vi "attoDllErrorHandler.vi"(6 "response":string, 9 "error in":errorcluster, 11 "rc":i32) -> (1 "error out":errorcluster)   [LabVIEW 2016]
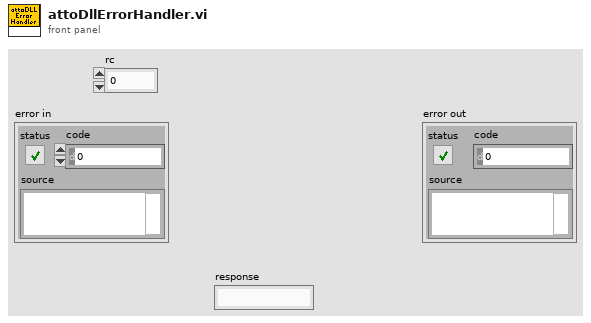
[diagram p1: front panel]
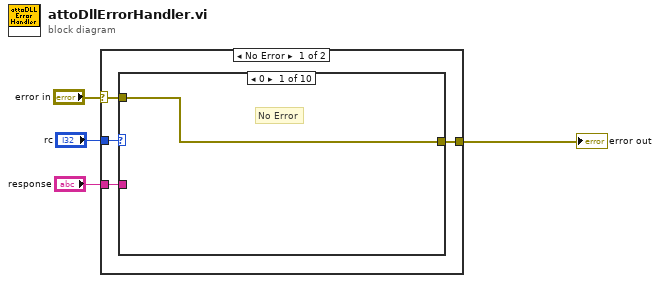
[diagram p0: block diagram]
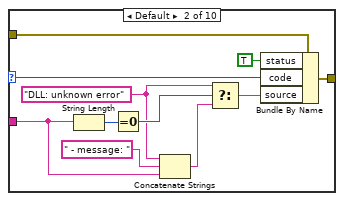
[diagram p2: hidden frame]
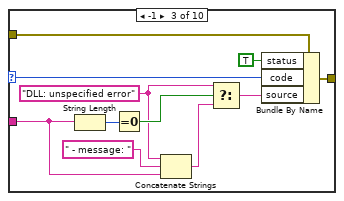
[diagram p3: hidden frame]
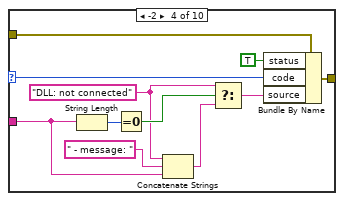
[diagram p4: hidden frame]
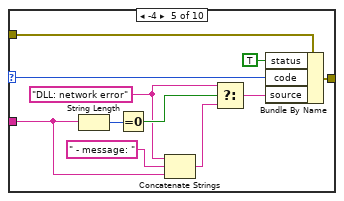
[diagram p5: hidden frame]
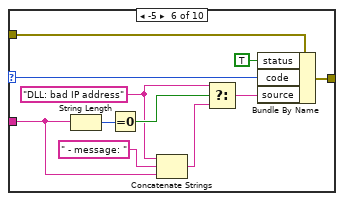
[diagram p6: hidden frame]
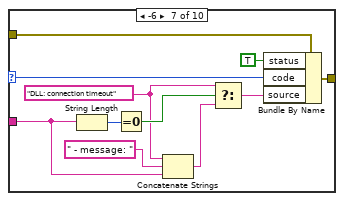
[diagram p7: hidden frame]
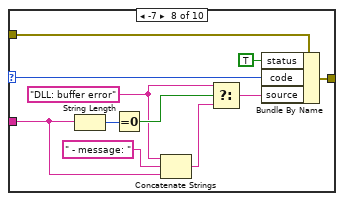
[diagram p8: hidden frame]
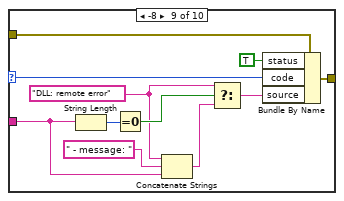
[diagram p9: hidden frame]
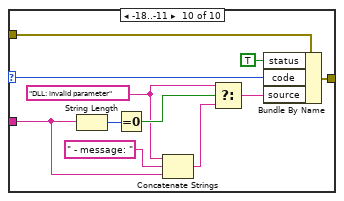
[diagram p10: hidden frame]
diagram:
  n1 = case shown="No Error" "error in" {
    selector: "error in" -> [w6 w109]
    tunnel: "rc" -> [w8 _]
    tunnel: [w7 w109] -> w2
    tunnel: "response" -> [w5 _]
    frame No Error {
      n2 = case shown="0" w8 {
        selector: w8 -> [_ w13 w24 w35 w46 w62 w65 w79 w90 w101]
        tunnel: [w9 w11 w22 w33 w44 w61 w69 w76 w88 w98] -> w7
        tunnel: w6 -> [w9 w14 w25 w36 w47 w63 w68 w80 w91 w102]
        tunnel: w5 -> [_ w12 w23 w34 w45 w56 w66 w78 w89 w100]
        frame 0 {
          # "No Error"
        }
        frame Default {
          w10 = "DLL: unknown error"
          n3 = String Length(string=w12) -> (length=w19:i32)
          n4 = Equal To 0?(x=w19) -> (x = 0?=w17:bool)
          n5 = Concatenate Strings(w10, " - message: " ("string"), w12) -> (w15:string)
          n6 = Select(t=w10, s=w17, f=w15) -> (s? t:f=w16:string)
          n7 = Bundle By Name(cluster=w14, "status"=TRUE, "code"=w13, "source"=w16) -> (w11:errorcluster)
        }
        frame -1 {
          w21 = "DLL: unspecified error"
          n8 = String Length(string=w23) -> (length=w30:i32)
          n9 = Equal To 0?(x=w30) -> (x = 0?=w28:bool)
          n10 = Concatenate Strings(w21, " - message: " ("string"), w23) -> (w26:string)
          n11 = Select(t=w21, s=w28, f=w26) -> (s? t:f=w27:string)
          n12 = Bundle By Name(cluster=w25, "status"=TRUE, "code"=w24, "source"=w27) -> (w22:errorcluster)
        }
        frame -2 {
          w32 = "DLL: not connected"
          n13 = String Length(string=w34) -> (length=w41:i32)
          n14 = Equal To 0?(x=w41) -> (x = 0?=w39:bool)
          n15 = Concatenate Strings(w32, " - message: " ("string"), w34) -> (w37:string)
          n16 = Select(t=w32, s=w39, f=w37) -> (s? t:f=w38:string)
          n17 = Bundle By Name(cluster=w36, "status"=TRUE, "code"=w35, "source"=w38) -> (w33:errorcluster)
        }
        frame -4 {
          w43 = "DLL: network error"
          n18 = String Length(string=w45) -> (length=w52:i32)
          n19 = Equal To 0?(x=w52) -> (x = 0?=w50:bool)
          n20 = Concatenate Strings(w43, " - message: " ("string"), w45) -> (w48:string)
          n21 = Select(t=w43, s=w50, f=w48) -> (s? t:f=w49:string)
          n22 = Bundle By Name(cluster=w47, "status"=TRUE, "code"=w46, "source"=w49) -> (w44:errorcluster)
        }
        frame -5 {
          w57 = "DLL: bad IP address"
          n23 = String Length(string=w56) -> (length=w60:i32)
          n24 = Equal To 0?(x=w60) -> (x = 0?=w58:bool)
          n25 = Concatenate Strings(w57, " - message: " ("string"), w56) -> (w54:string)
          n26 = Select(t=w57, s=w58, f=w54) -> (s? t:f=w55:string)
          n27 = Bundle By Name(cluster=w63, "status"=TRUE, "code"=w62, "source"=w55) -> (w61:errorcluster)
        }
        frame -6 {
          w67 = "DLL: connection timeout"
          n28 = String Length(string=w66) -> (length=w74:i32)
          n29 = Equal To 0?(x=w74) -> (x = 0?=w72:bool)
          n30 = Concatenate Strings(w67, " - message: " ("string"), w66) -> (w70:string)
          n31 = Select(t=w67, s=w72, f=w70) -> (s? t:f=w71:string)
          n32 = Bundle By Name(cluster=w68, "status"=TRUE, "code"=w65, "source"=w71) -> (w69:errorcluster)
        }
        frame -7 {
          w77 = "DLL: buffer error"
          n33 = String Length(string=w78) -> (length=w85:i32)
          n34 = Equal To 0?(x=w85) -> (x = 0?=w83:bool)
          n35 = Concatenate Strings(w77, " - message: " ("string"), w78) -> (w81:string)
          n36 = Select(t=w77, s=w83, f=w81) -> (s? t:f=w82:string)
          n37 = Bundle By Name(cluster=w80, "status"=TRUE, "code"=w79, "source"=w82) -> (w76:errorcluster)
        }
        frame -8 {
          w87 = "DLL: remote error"
          n38 = String Length(string=w89) -> (length=w96:i32)
          n39 = Equal To 0?(x=w96) -> (x = 0?=w94:bool)
          n40 = Concatenate Strings(w87, " - message: " ("string"), w89) -> (w92:string)
          n41 = Select(t=w87, s=w94, f=w92) -> (s? t:f=w93:string)
          n42 = Bundle By Name(cluster=w91, "status"=TRUE, "code"=w90, "source"=w93) -> (w88:errorcluster)
        }
        frame -18..-11 {
          w99 = "DLL: invalid parameter"
          n43 = String Length(string=w100) -> (length=w107:i32)
          n44 = Equal To 0?(x=w107) -> (x = 0?=w105:bool)
          n45 = Concatenate Strings(w99, " - message: " ("string"), w100) -> (w103:string)
          n46 = Select(t=w99, s=w105, f=w103) -> (s? t:f=w104:string)
          n47 = Bundle By Name(cluster=w102, "status"=TRUE, "code"=w101, "source"=w104) -> (w98:errorcluster)
        }
      }
    }
    frame Error {
    }
  }
  "error out" <- w2
